vi "Go Forward.vi"(8 "error in (no error)":errorcluster, 11 "WebView2 Control in":refnum<class "WebView2 Control.lvclass">) -> (0 "error out":errorcluster, 3 "WebView2 Control out":refnum<class "WebView2 Control.lvclass">)   [LabVIEW 2020, in "WebView2.lvlib" / "WebView2 Control.lvclass"]
uses:
  WebView2 Control.lvclass
  WebView2 Control.lvclass/WebView2 Control.ctl
  C:/Users/Simon/Documents/GitHub/LV-WebView2/Source/Libs/Microsoft.Web.WebView2.Core.dll
  Libs/Microsoft.Web.WebView2.Core.dll
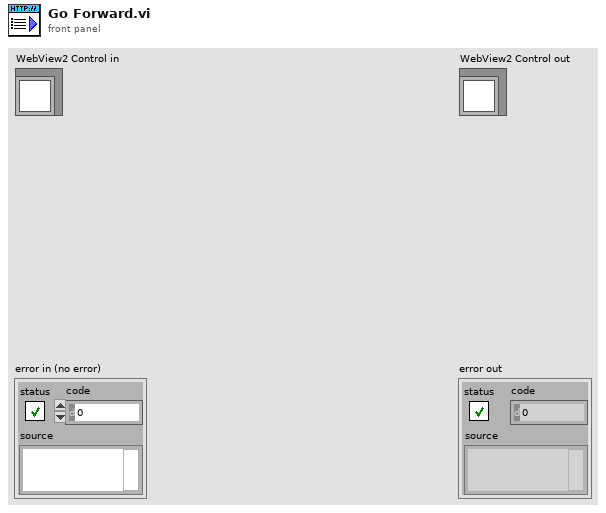
[diagram p1: front panel]
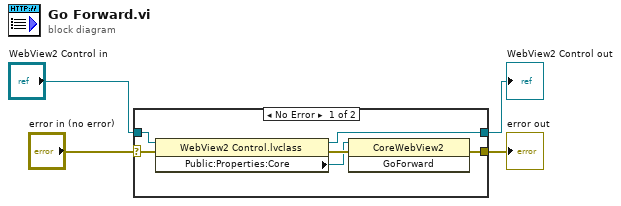
[diagram p0: block diagram]
diagram:
  n1 = case shown="No Error" "error in (no error)" {
    selector: "error in (no error)" -> [w10 w12]
    tunnel: [w6 w12] -> w3
    tunnel: [w7 w11] -> w1
    tunnel: "WebView2 Control in" -> [w8 w11]
    frame No Error {
      n2 = property class="WebView2 Control.lvclass"(reference=w8, error in=w10) -> (reference out=w7:refnum<class "WebView2 Control.lvclass">, error out=w9:errorcluster, "Public:Properties:Core"=w5:refnum<k24>)
      n3 = invoke class="CoreWebView2" method="GoForward"(reference=w5, error in=w9) -> (error out=w6:errorcluster)  [unwired: 1 in, 2 out]
    }
    frame Error {
    }
  }
  "error out" <- w3
  "WebView2 Control out" <- w1
